vi "GetDAC.vi"(0 "Number of DAC":T1 items=["DAC 1", "DAC 2", "DAC 3", "DAC 4"], 5 "error in":T2) -> (14 "DAC out":sgl format="%#_g V", 19 "error out":T2)   [LabVIEW 2016]
doc: "Returns the value at the DAC specified by 'Number of DAC', which is a required input."
uses:
  Controls/Error_Out.ctl
  Controls/DAC_Selection.ctl
  Files_ASC500/DLL/ASC500_RemoteControlV27.dll
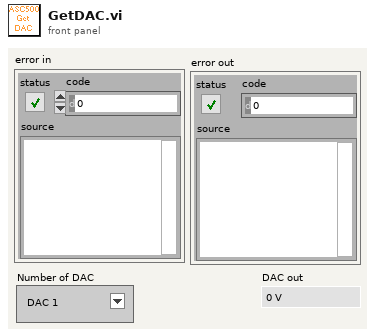
[diagram p1: front panel]
types:
  T1 = typedef "DAC_Selection.ctl" = u16
  T2 = typedef "Error_Out.ctl" = errorcluster
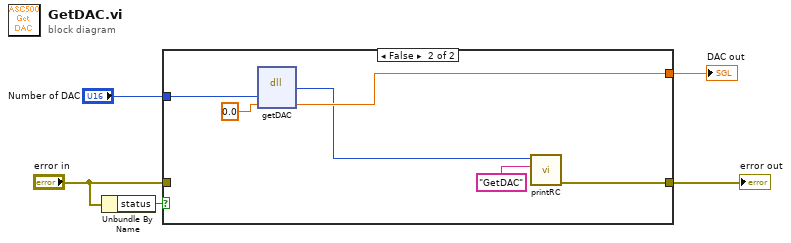
[diagram p0: block diagram]
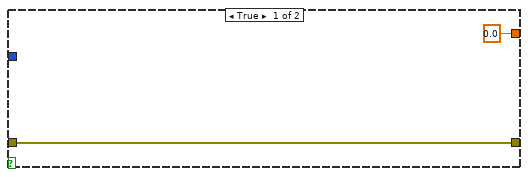
[diagram p2: hidden frame]
diagram:
  n1 = Unbundle By Name("error in") -> ("status"=w4:bool)
  n2 = case shown="False" w4 {
    tunnel: [w6 w9] -> w2
    tunnel: "Number of DAC" -> [_ w12]
    tunnel: [sgl 0.0 ("Value") w11] -> w5
    tunnel: "error in" -> [w6 _]
    frame True {
    }
    frame False {
      n3 = dll-call lib="G:/SCMOperations/Share/ELE/Produkt Information/ASC500/04 Remote Control/02 development versions/2018Nov06/Files_ASC500/DLL/ASC500_RemoteControlV27.dll" fn="getDAC"("Number"=w12, "Value"=sgl 0.0) -> ("return type"=w8:i32, "Value"=w11:sgl)  [unwired: 4 in, 2 out]
      n4 = call "printRC.vi"("additional information"="GetDAC", "RC"=w8) -> ("error out"=w9:T2)  [unwired: 9 in]
    }
  }
  "error out" <- w2
  "DAC out" <- w5
